vi "test.vi"() -> ()   [LabVIEW 2017]
panel:
  out "joystick info":T1(array[cluster])
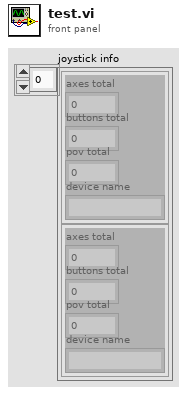
[diagram p1: front panel]
types:
  T1 = cluster{"axes total":u32, "buttons total":u32, "pov total":u32, "device name":string}[]
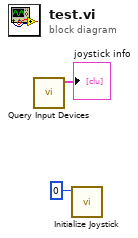
[diagram p0: block diagram]
diagram:
  n1 = call <vilib>:"Query Input Devices.vi"() -> ("joystick info"=→"joystick info":T1)  [unwired: 8 in, 3 out]
  n2 = call <vilib>:"Initialize Joystick.vi"("device index"=0) -> ()  [unwired: 9 in, 2 out]
